vi "Configure Marker Search.vi"(7 "Marker Search":T1(ring), 8 "error in (no error)":errorcluster, 9 "Target Value":dbl, 10 "Marker Number":u8=1, 11 "VNA-FieldFox in":refnum<class "VNA-FieldFox.lvclass">) -> (0 "error out":errorcluster, 3 "VNA-FieldFox out":refnum<class "VNA-FieldFox.lvclass">)   [LabVIEW 2020, in "VNA-FieldFox.lvclass"]
doc: "Configures and excecutes a marker search.\nThe marker is on the active trace."
uses:
  VNA-FieldFox.lvclass
  Vector Network Analyzer.lvclass
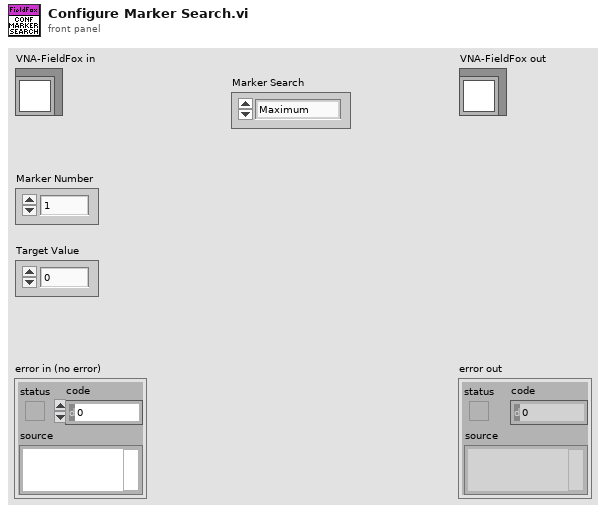
[diagram p1: front panel]
types:
  T1 = enum16{"Maximum", "Minimum", "Right Peak", "Left Peak", "Negative Peak", "Taget Value", "Left Taget Value", "Rigth Target Value"}
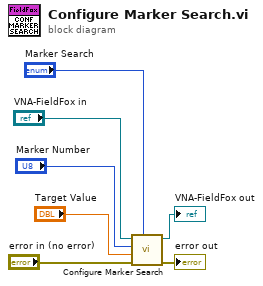
[diagram p0: block diagram]
diagram:
  n1 = call-parent "Configure Marker Search.vi"("Marker Search"="Marker Search", "error in (no error)"="error in (no error)", "Target Value"="Target Value", "Marker Number"="Marker Number", "Vector Network Analyzer in"="VNA-FieldFox in") -> ("error out"=→"error out":errorcluster, "Vector Network Analyzer out"=→"VNA-FieldFox out":refnum<class "VNA-FieldFox.lvclass">)  [unwired: 5 in]
